vi "Write moduleName.vi"(8 "error in (no error)":errorcluster, 10 "moduleName":string, 11 "Enumeration in":refnum<class "Enumeration.lvclass">) -> (0 "error out":errorcluster, 3 "Enumeration out":refnum<class "Enumeration.lvclass">)   [LabVIEW 2016, in "Enumeration.lvclass"]
uses:
  Enumeration.lvclass
  Enumeration.lvclass/Enumeration.ctl
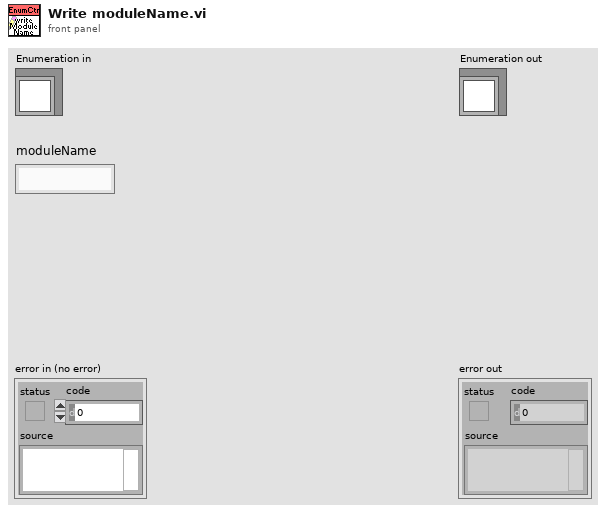
[diagram p1: front panel]
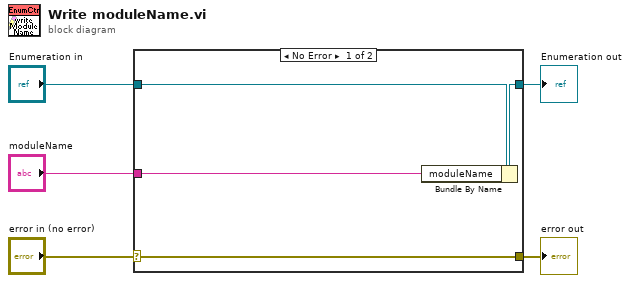
[diagram p0: block diagram]
diagram:
  n1 = case shown="No Error" "error in (no error)" {
    selector: "error in (no error)" -> [w9 w10]
    tunnel: [w9 w10] -> w4
    tunnel: [w7 w11] -> w2
    tunnel: "Enumeration in" -> [w8 w11]
    tunnel: "moduleName" -> [w6 _]
    frame No Error {
      n2 = Bundle By Name(cluster=w8, "moduleName"=w6) -> (w7:refnum<class "Enumeration.lvclass">)
    }
    frame Error {
    }
  }
  "error out" <- w4
  "Enumeration out" <- w2
